vi "Copy自定义数据.vi"() -> ()   [LabVIEW 2018]
uses:
  <vilib>/vision/Image Controls.llb/IMAQ Image.ctl
panel:
  out "Image Dst Out":T1
  out "Custom Data Out":string
  in  "路径":path
  out "error out":errorcluster
  in  "error in (no error)":errorcluster
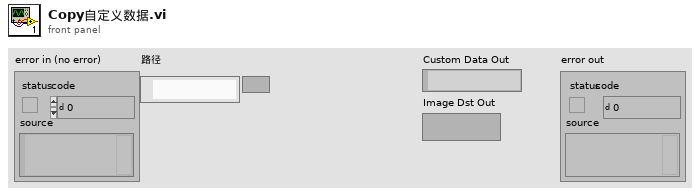
[diagram p1: front panel]
types:
  T1 = typedef "IMAQ Image.ctl" = refnum<image>
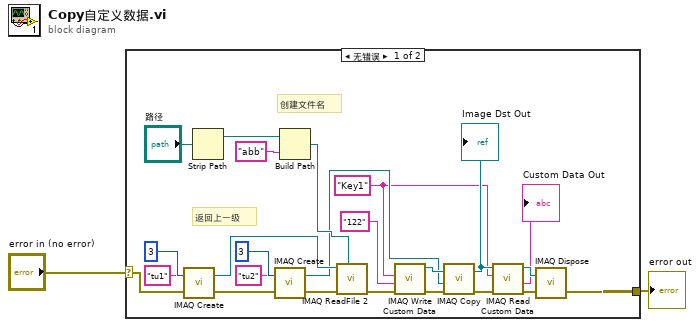
[diagram p0: block diagram]
diagram:
  n1 = case shown="无错误" "error in (no error)" {
    selector: "error in (no error)" -> [w4 w27]
    tunnel: [w26 w27] -> w2
    frame No Error {
      w8 = "Key1" ("Key")
      # "创建文件名"
      # "返回上一级"
      n2 = call "IMAQ Create"("Border Size"=3, "Image Name"="tu1", "error in (no error)"=w4) -> ("New Image"=w16:T1, "error out"=w25:errorcluster)  [unwired: 2 in]
      n3 = Strip Path(path="路径") -> (stripped path=w20:path)  [unwired: 1 out]
      n4 = call "IMAQ Create"("Border Size"=3, "Image Name"="tu2", "error in (no error)"=w25) -> ("New Image"=w10:T1, "error out"=w15:errorcluster)  [unwired: 2 in]
      n5 = Build Path(base path=w20, name or relative path="abb" ("名称或相对路径")) -> (appended path=w17:path)
      n6 = call "IMAQ ReadFile 2"("File Path"=w17, "error in (no error)"=w15, "Image"=w16) -> ("error out"=w13:errorcluster)  [unwired: 4 in, 4 out]
      n7 = call "IMAQ Write Custom Data"("error in (no error)"=w13, "Custom Data In"="122", "Key"=w8) -> ("error out"=w11:errorcluster, "Image Out"=w12:T1)  [unwired: 7 in]
      n8 = call "IMAQ Copy"("error in (no error)"=w11, "Image Dst"=w10, "Image Src"=w12) -> ("error out"=w7:errorcluster, "Image Dst Out"=w9:T1)  [unwired: 3 in]
      "Image Dst Out" <- w9
      n9 = call "IMAQ Read Custom Data"("error in (no error)"=w7, "Key"=w8, "Image"=w9) -> ("error out"=w5:errorcluster, "Custom Data Out"=→"Custom Data Out":string, "Image (duplicate)"=w6:T1)  [unwired: 6 in]
      n10 = call "IMAQ Dispose"("Image"=w6, "error in (no error)"=w5) -> ("error out"=w26:errorcluster)  [unwired: 4 in]
    }
    frame Error {
    }
  }
  "error out" <- w2
